vi "Enqueue Enum (array).vi"(7 "Place at beginning (F)":bool[](array[boolean]), 8 "error in":errorcluster, 9 "Data":variant[](array[variant]), 10 "States":i32[](array[numeric]), 11 "Queue In":refnum<queue>) -> (0 "error out":errorcluster, 3 "Queue Out":refnum<queue>)   [LabVIEW 2020, in "Enum Queue State Machine.lvlib"]
uses:
  Enum Queue State Machine.lvlib
  Controls/Enum Message.ctl
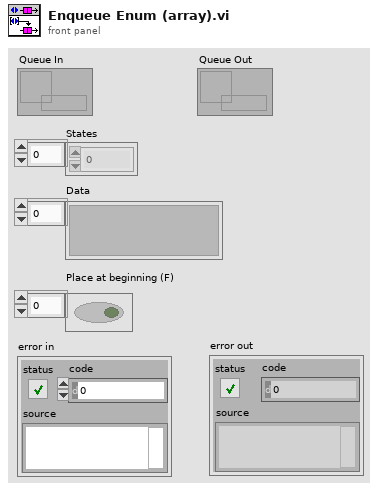
[diagram p1: front panel]
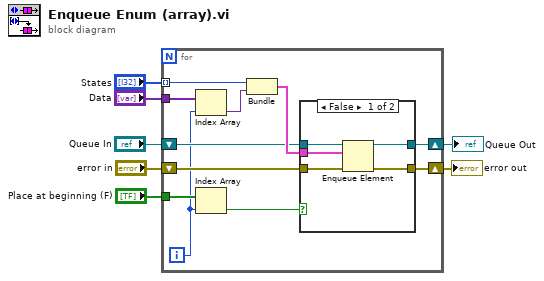
[diagram p0: block diagram]
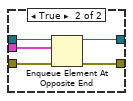
[diagram p2: hidden frame]
diagram:
  n1 = for {
    tunnel: "Place at beginning (F)" -> [w12]
    tunnel: "States" -> [w15] mode=indexing
    tunnel: "Data" -> [w9]
    shift-right: [w17] -> w6
    shift-left: "error in" -> [w18]
    shift-right: [w14] -> w1
    shift-left: "Queue In" -> [w13]
    i -> [w8]
    n2 = Index Array(array=w9, index=w8) -> (element=w10:variant)
    n3 = Index Array(array=w12, index=w8) -> (element=w11:bool)
    n4 = Bundle("State"=w15, "Data"=w10) -> (w16:cluster{"State":i32, "Data":variant})  [unwired: 1 in]
    n5 = case shown="False" w11 {
      tunnel: w18 -> [w21 w28]
      tunnel: [w20 w27] -> w17
      tunnel: w13 -> [w23 w26]
      tunnel: [w22 w25] -> w14
      tunnel: w16 -> [w19 w24]
      frame False {
        n6 = Enqueue Element(queue=w23, element=w19, error in (no error)=w21) -> (queue out=w22:refnum<queue>, error out=w20:errorcluster)  [unwired: 1 in, 1 out]
      }
      frame True {
        n7 = Enqueue Element At Opposite End(queue=w26, element=w24, error in (no error)=w28) -> (queue out=w25:refnum<queue>, error out=w27:errorcluster)  [unwired: 1 in, 1 out]
      }
    }
  }
  "error out" <- w6
  "Queue Out" <- w1
